vi "Format RF Power String.vi"(11 "x":dbl) -> (3 "result string":string)   [LabVIEW 2018, in "Power Sweep.lvlib" / "Power Sweep.lvclass"]
uses:
  Power Sweep.lvclass
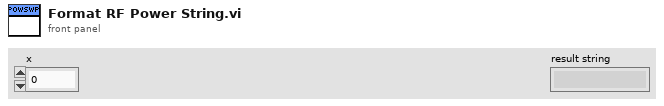
[diagram p1: front panel]
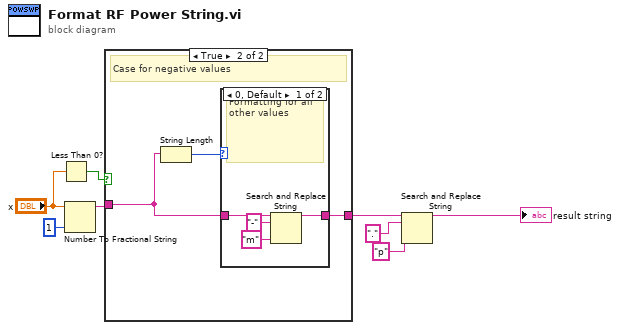
[diagram p0: block diagram]
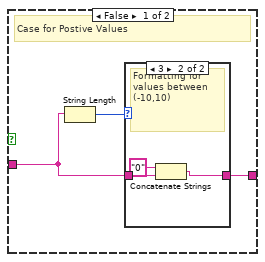
[diagram p2: hidden frame]
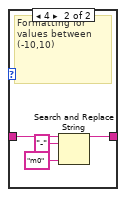
[diagram p4: hidden frame]
diagram:
  n1 = Less Than 0?(x="x") -> (x < 0?=w3:bool)
  n2 = Number To Fractional String(number="x", precision (6)=i16 1) -> (F-format string=w2:string)  [unwired: 2 in]
  n3 = case shown="True" w3 {
    tunnel: [w10 w17] -> w6
    tunnel: w2 -> [w9 w16]
    frame False {
      # "Case for Postive Values"
      n4 = String Length(string=w9) -> (length=w11:i32)
      n5 = case shown="3" w11 {
        tunnel: w9 -> [w12 w14]
        tunnel: [w12 w15] -> w10
        frame 0, Default {
          # "no formatting necessary for all other values"
        }
        frame 3 {
          # "Formatting for values between (-10,10)"
          n6 = Concatenate Strings("0" ("string"), w14) -> (w15:string)
        }
      }
    }
    frame True {
      # "Case for negative values"
      n7 = String Length(string=w16) -> (length=w18:i32)
      n8 = case shown="0, Default" w18 {
        tunnel: w16 -> [w21 w25]
        tunnel: [w22 w26] -> w17
        frame 0, Default {
          # "Formatting for all other values"
          n9 = Search and Replace String(input string=w21, search string="-", replace string="m" ("replace string (\"\")")) -> (result string=w22:string)  [unwired: 5 in, 3 out]
        }
        frame 4 {
          # "Formatting for values between (-10,10)"
          n10 = Search and Replace String(input string=w25, search string="-", replace string="m0" ("replace string (\"\")")) -> (result string=w26:string)  [unwired: 5 in, 3 out]
        }
      }
    }
  }
  n11 = Search and Replace String(input string=w6, search string=".", replace string="p" ("replace string (\"\")")) -> (result string=→"result string":string)  [unwired: 5 in, 3 out]
